vi "setting.vi"() -> ()   [LabVIEW 2019, in "Setting Lib.lvlib"]
uses:
  Setting Lib.lvlib
  User Lib.lvlib
  Calibration Lib.lvlib
  database.lvlib
panel:
  out "Error out 4":errorcluster
  in  "Error in 2":errorcluster
  out "Error out 3":errorcluster
  out "Error out 2":errorcluster
  out "Error out":errorcluster
  out "String":string
  in  "Close":bool
  in  "Calibration":bool
  in  "General":bool
  in  "Speed Control":bool
  in  "User":bool
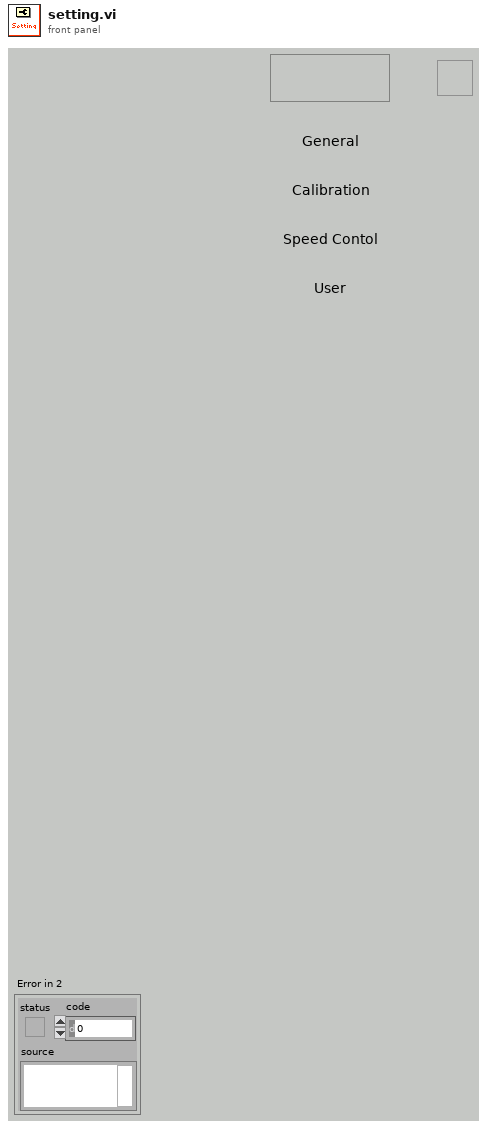
[diagram p1: front panel]
types:
  T1 = cluster{string, "date/time string":string, "date/time string":string, string}
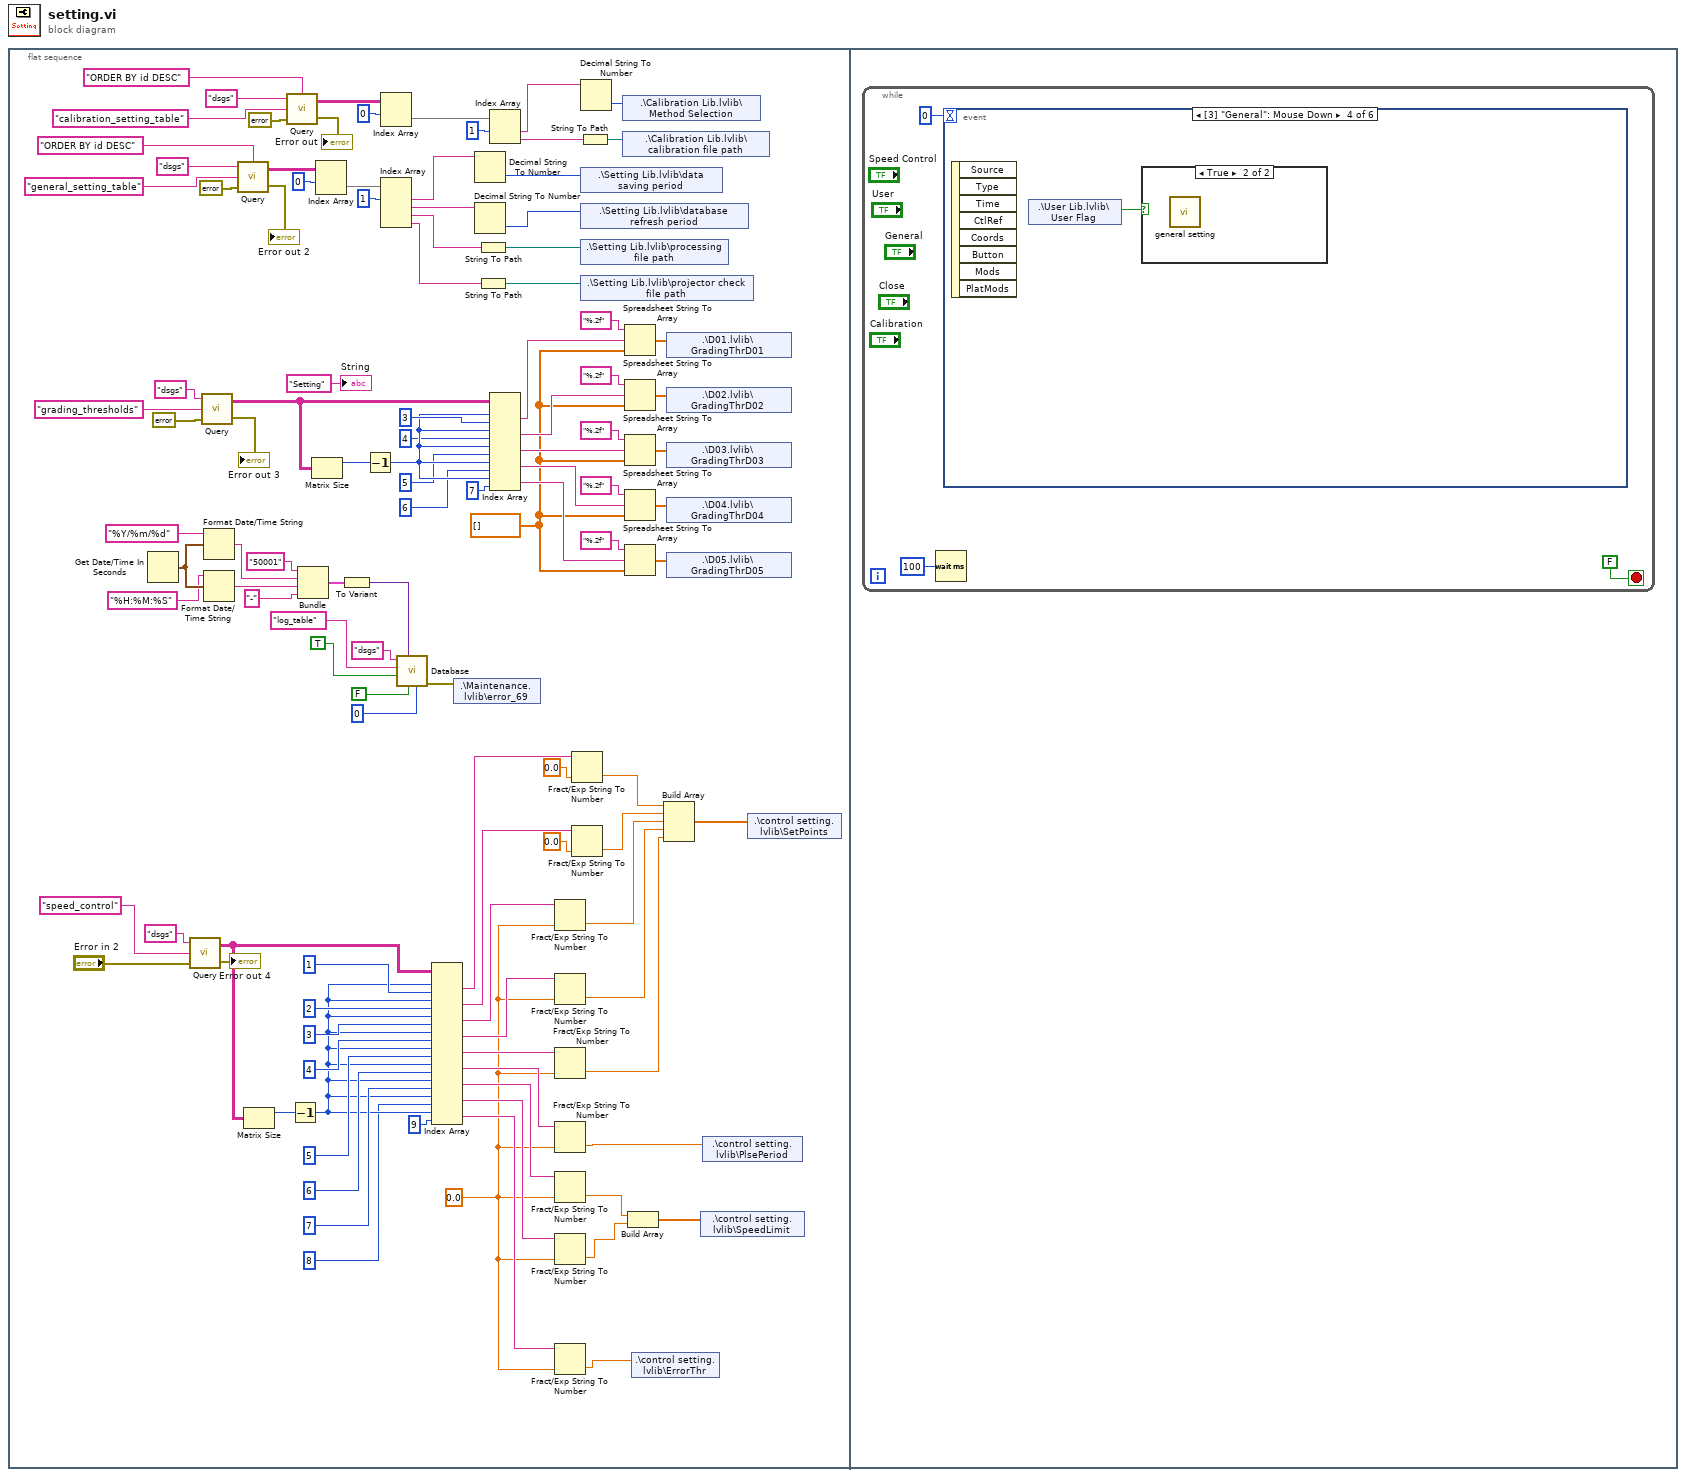
[diagram p0: block diagram]
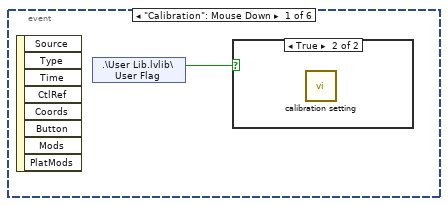
[diagram p2: hidden frame]
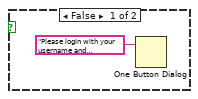
[diagram p3: hidden frame]
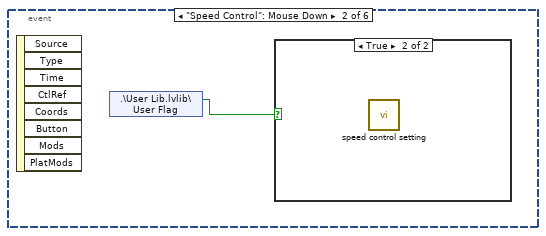
[diagram p4: hidden frame]
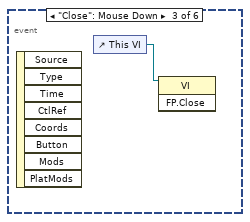
[diagram p6: hidden frame]
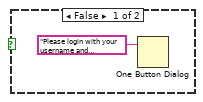
[diagram p7: hidden frame]
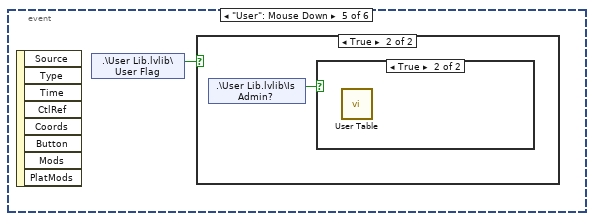
[diagram p8: hidden frame]
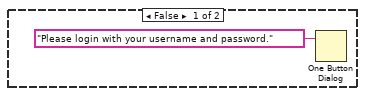
[diagram p9: hidden frame]
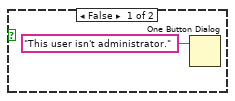
[diagram p10: hidden frame]
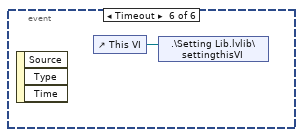
[diagram p11: hidden frame]
diagram:
  n1 = flat-sequence {
    frame #0 {
      w13 = 0.0 ("default (0 DBL)")
      w93 = dbl[] []
      n2 = Get Date/Time In Seconds() -> (seconds since 1Jan1904=w51:timestamp)
      n3 = call "Query.vi"("Error in"="Error in 2", "Table Name"="speed_control", "Connection Name"="dsgs") -> ("Error out"=→"Error out 4":errorcluster, "data"=w18:string[][])  [unwired: 1 in]
      n4 = call "Query.vi"("Error in"=errorcluster {"status"=FALSE, "code"=0, "source"=""}, "Table Name"="grading_thresholds", "Connection Name"="dsgs") -> ("Error out"=→"Error out 3":errorcluster, "data"=w111:string[][])  [unwired: 1 in]
      n5 = Format Date/Time String(time format string (%c)="%Y/%m/%d", seconds (now)=w51) -> (date/time string=w48:string)  [unwired: 1 in]
      n6 = Format Date/Time String(time format string (%c)="%H:%M:%S", seconds (now)=w51) -> (date/time string=w47:string)  [unwired: 1 in]
      n7 = call "Query.vi"("Condition"="ORDER BY id DESC", "Error in"=errorcluster {"status"=FALSE, "code"=0, "source"=""}, "Table Name"="general_setting_table", "Connection Name"="dsgs") -> ("Error out"=→"Error out 2":errorcluster, "data"=w82:string[][])
      n8 = Matrix Size(0:w18) -> (1:w36:i32)  [unwired: 1 out]
      n9 = call "Query.vi"("Condition"="ORDER BY id DESC", "Error in"=errorcluster {"status"=FALSE, "code"=0, "source"=""}, "Table Name"="calibration_setting_table", "Connection Name"="dsgs") -> ("Error out"=→"Error out":errorcluster, "data"=w64:string[][])
      n10 = Decrement(x=w36) -> (x-1=w28:i32)
      n11 = Bundle("50001", "date/time string"=w48, "date/time string"=w47, "-") -> (w45:T1)  [unwired: 1 in]
      n12 = Matrix Size(0:w111) -> (1:w110:i32)  [unwired: 1 out]
      n13 = Index Array(array=w82, index (row)=0) -> (element=w80:string[])  [unwired: 1 in]
      n14 = To Variant(anything=w45) -> (Variant=w44:variant)
      n15 = Decrement(x=w110) -> (x-1=w108:i32)
      n16 = Index Array(array=w64, index (row)=0) -> (element=w66:string[])  [unwired: 1 in]
      n17 = Index Array(array=w80, index #1=1 ("index")) -> (element #1=w78:string, element #2=w77:string, element #3=w76:string, element #4=w75:string)  [unwired: 3 in]
      n18 = call "Database.vi"("Maximum Row"=u64 0 ("Storage Time (Day)"), "Delete row?"=FALSE, "Data"=w44, "Auto Increment ID?"=TRUE, "Table"="log_table", "Connection"="dsgs") -> ("Error out"=w40:errorcluster)  [unwired: 5 in]
      n19 = Index Array(array=w18, index (row) #1=w28, index (col) #1=1 ("disabled index (col)"), index (row) #2=w28, index (col) #2=2 ("disabled index (col)"), index (row) #3=w28, index (col) #3=3 ("disabled index (col)"), index (row) #4=w28, index (col) #4=4 ("disabled index (col)"), index (row) #5=w28, index (col) #5=5 ("disabled index (col)"), index (row) #6=w28, index (col) #6=6 ("disabled index (col)"), index (row) #7=w28, index (col) #7=7 ("disabled index (col)"), index (row) #8=w28, index (col) #8=8 ("disabled index (col)"), index (row) #9=w28, index (col) #9=9 ("disabled index (col)")) -> (element #1=w25:string, element #2=w22:string, element #3=w21:string, element #4=w20:string, element #5=w19:string, element #6=w17:string, element #7=w16:string, element #8=w15:string, element #9=w14:string)
      n20 = shared-variable ".\\Maintenance.lvlib\\error_69"(w40) -> ()  [unwired: 1 in, 1 out]
      n21 = Decimal String To Number(string=w78) -> (number=w71:i32)  [unwired: 2 in, 1 out]
      n22 = Decimal String To Number(string=w77) -> (number=w72:i32)  [unwired: 2 in, 1 out]
      n23 = String To Path(string=w76) -> (path=w73:path)
      n24 = String To Path(string=w75) -> (path=w74:path)
      n25 = Index Array(array=w66, index #1=1 ("index")) -> (element #1=w68:string, element #2=w59:string)  [unwired: 1 in]
      n26 = Index Array(array=w111, index (row) #1=w108, index (col) #1=3 ("disabled index (col)"), index (row) #2=w108, index (col) #2=4 ("disabled index (col)"), index (row) #3=w108, index (col) #3=5 ("disabled index (col)"), index (row) #4=w108, index (col) #4=6 ("disabled index (col)"), index (row) #5=w108, index (col) #5=7 ("disabled index (col)")) -> (element #1=w103:string, element #2=w97:string, element #3=w96:string, element #4=w95:string, element #5=w94:string)
      n27 = Fract/Exp String To Number(string=w21, default (0 dbl)=w13) -> (number=w10:dbl)  [unwired: 2 in, 1 out]
      n28 = Fract/Exp String To Number(string=w20, default (0 dbl)=w13) -> (number=w9:dbl)  [unwired: 2 in, 1 out]
      n29 = Fract/Exp String To Number(string=w19, default (0 dbl)=w13) -> (number=w8:dbl)  [unwired: 2 in, 1 out]
      n30 = Fract/Exp String To Number(string=w17, default (0 dbl)=w13) -> (number=w6:dbl)  [unwired: 2 in, 1 out]
      n31 = Fract/Exp String To Number(string=w16, default (0 dbl)=w13) -> (number=w5:dbl)  [unwired: 2 in, 1 out]
      n32 = Fract/Exp String To Number(string=w15, default (0 dbl)=w13) -> (number=w4:dbl)  [unwired: 2 in, 1 out]
      n33 = Fract/Exp String To Number(string=w14, default (0 dbl)=w13) -> (number=w2:dbl)  [unwired: 2 in, 1 out]
      n34 = Fract/Exp String To Number(string=w25, default (0 dbl)=0.0 ("default (0 DBL)")) -> (number=w12:dbl)  [unwired: 2 in, 1 out]
      n35 = Fract/Exp String To Number(string=w22, default (0 dbl)=0.0 ("default (0 DBL)")) -> (number=w11:dbl)  [unwired: 2 in, 1 out]
      n36 = String To Path(string=w59) -> (path=w69:path)
      n37 = Decimal String To Number(string=w68) -> (number=w70:i32)  [unwired: 2 in, 1 out]
      n38 = shared-variable ".\\Setting Lib.lvlib\\data saving period"(w71) -> ()  [unwired: 1 in, 1 out]
      n39 = shared-variable ".\\Setting Lib.lvlib\\database refresh period"(w72) -> ()  [unwired: 1 in, 1 out]
      n40 = shared-variable ".\\Setting Lib.lvlib\\processing file path"(w73) -> ()  [unwired: 1 in, 1 out]
      n41 = shared-variable ".\\Setting Lib.lvlib\\projector check file path"(w74) -> ()  [unwired: 1 in, 1 out]
      n42 = shared-variable ".\\Calibration Lib.lvlib\\Method Selection"(w70) -> ()  [unwired: 1 in, 1 out]
      n43 = shared-variable ".\\Calibration Lib.lvlib\\calibration file path"(w69) -> ()  [unwired: 1 in, 1 out]
      n44 = Spreadsheet String To Array(format string="%.2f", spreadsheet string=w103, array type (2D Dbl)=w93) -> (array=w92:dbl[])  [unwired: 1 in]
      n45 = Spreadsheet String To Array(format string="%.2f", spreadsheet string=w97, array type (2D Dbl)=w93) -> (array=w91:dbl[])  [unwired: 1 in]
      n46 = Spreadsheet String To Array(format string="%.2f", spreadsheet string=w96, array type (2D Dbl)=w93) -> (array=w90:dbl[])  [unwired: 1 in]
      n47 = Spreadsheet String To Array(format string="%.2f", spreadsheet string=w95, array type (2D Dbl)=w93) -> (array=w89:dbl[])  [unwired: 1 in]
      n48 = Spreadsheet String To Array(format string="%.2f", spreadsheet string=w94, array type (2D Dbl)=w93) -> (array=w88:dbl[])  [unwired: 1 in]
      n49 = Build Array(w5, w4) -> (w3:dbl[])
      n50 = shared-variable ".\\control setting.lvlib\\ErrorThr"(w2) -> ()  [unwired: 1 in, 1 out]
      n51 = Build Array(w12, w11, w10, w9, w8) -> (w7:dbl[])
      n52 = shared-variable ".\\D01.lvlib\\GradingThrD01"(w92) -> ()  [unwired: 1 in, 1 out]
      n53 = shared-variable ".\\D02.lvlib\\GradingThrD02"(w91) -> ()  [unwired: 1 in, 1 out]
      n54 = shared-variable ".\\D03.lvlib\\GradingThrD03"(w90) -> ()  [unwired: 1 in, 1 out]
      n55 = shared-variable ".\\D04.lvlib\\GradingThrD04"(w89) -> ()  [unwired: 1 in, 1 out]
      n56 = shared-variable ".\\D05.lvlib\\GradingThrD05"(w88) -> ()  [unwired: 1 in, 1 out]
      n57 = shared-variable ".\\control setting.lvlib\\SpeedLimit"(w3) -> ()  [unwired: 1 in, 1 out]
      n58 = shared-variable ".\\control setting.lvlib\\PlsePeriod"(w6) -> ()  [unwired: 1 in, 1 out]
      n59 = shared-variable ".\\control setting.lvlib\\SetPoints"(w7) -> ()  [unwired: 1 in, 1 out]
      "String" <- "Setting" ("String")
    }
    frame #1 {
      n60 = while {
        stop <- FALSE stop-if-true
        n61 = Wait (ms)(milliseconds to wait=u32 100) -> ()  [unwired: 1 out]
        n62 = event shown="[3] \"General\": Mouse Down" {
          selector: _ -> [_ _ _ _ _ _]
          dyn-events: _ -> [_ _ _ _ _ _]
          timeout: 0 -> [_ _ _ _ _ _]
          event "Calibration": Mouse Down {
            n63 = event-data() -> ()  [unwired: 1 in, 8 out]
            n64 = shared-variable ".\\User Lib.lvlib\\User Flag"() -> (w117:bool)  [unwired: 1 in, 1 out]
            n65 = case shown="True" w117 {
              frame False {
                n66 = One Button Dialog(message="Please login with your username and password.") -> ()  [unwired: 1 in, 1 out]
              }
              frame True {
                n67 = call "calibration setting.vi"() -> ()  [unwired: 12 in]
              }
            }
          }
          event "Speed Control": Mouse Down {
            n68 = event-data() -> ()  [unwired: 1 in, 8 out]
            n69 = shared-variable ".\\User Lib.lvlib\\User Flag"() -> (w119:bool)  [unwired: 1 in, 1 out]
            n70 = case shown="True" w119 {
              frame False {
              }
              frame True {
                n71 = call "speed control setting.vi"() -> ()  [unwired: 12 in]
              }
            }
          }
          event "Close": Mouse Down {
            n72 = event-data() -> ()  [unwired: 1 in, 8 out]
            n73 = control-ref of="This VI"() -> (w120:refnum<vi>)
            n74 = invoke class="VI" method="FP.Close"(reference=w120) -> ()  [unwired: 2 in, 3 out]
          }
          event "General": Mouse Down {
            n75 = event-data() -> ()  [unwired: 1 in, 8 out]
            n76 = shared-variable ".\\User Lib.lvlib\\User Flag"() -> (w121:bool)  [unwired: 1 in, 1 out]
            n77 = case shown="True" w121 {
              frame False {
                n78 = One Button Dialog(message="Please login with your username and password.") -> ()  [unwired: 1 in, 1 out]
              }
              frame True {
                n79 = call "general setting.vi"() -> ()  [unwired: 12 in]
              }
            }
          }
          event "User": Mouse Down {
            n80 = event-data() -> ()  [unwired: 1 in, 8 out]
            n81 = shared-variable ".\\User Lib.lvlib\\User Flag"() -> (w123:bool)  [unwired: 1 in, 1 out]
            n82 = case shown="True" w123 {
              frame False {
                n83 = One Button Dialog(message="Please login with your username and password.") -> ()  [unwired: 1 in, 1 out]
              }
              frame True {
                n84 = shared-variable ".\\User Lib.lvlib\\Is Admin?"() -> (w125:bool)  [unwired: 1 in, 1 out]
                n85 = case shown="True" w125 {
                  frame False {
                    n86 = One Button Dialog(message="This user isn't administrator.") -> ()  [unwired: 1 in, 1 out]
                  }
                  frame True {
                    n87 = call "User Table.vi"() -> ()  [unwired: 12 in]
                  }
                }
              }
            }
          }
          event Timeout {
            n88 = event-data() -> ()  [unwired: 1 in, 3 out]
            n89 = control-ref of="This VI"() -> (w127:refnum<vi>)
            n90 = shared-variable ".\\Setting Lib.lvlib\\settingthisVI"(w127) -> ()  [unwired: 1 in, 1 out]
          }
        }
      }
    }
  }
